vi "总磷插入数据.vi"(0 "table":string, 5 "data":T2={"时间标识"=timestamp(0 s since 1904-01-01), "测量模式"=enum."水样测试", "数据标记表"="N", "监测值"=0.0, "单位"=0, "数据标识"="", "因子编码"=0, "标样参考值"=0.0, "F0"=0.0, "F1"=0.0, "F2"=0.0, "F3"=0.0, "F4"=0.0, "F5"=0.0, "F6"=0.0, "F7"=0.0, "X"=0.0, "温度"=0.0, "湿度"=0.0, "量程标识"="", "SN"=""} {"单位" items=["μg/L", "mg/L", "ppm", "mg/m3", "cm", "ppb", "μg/m3", "%", "nmol/mol", "μmol/mol", "MPN/L", "MPN/100ml", "ng/m3", "NTU", "无量纲", "ms/cm", "μs/cm"]}, 11 "error in (no error)":errorcluster) -> (15 "error out":errorcluster)   [LabVIEW 2016, in "斯坦道总磷.lvlib"]
uses:
  <vilib>/Utility/sysdir.llb/System Directory Type.ctl
  <vilib>/Utility/error.llb/DialogType.ctl
  <vilib>/addons/database/Auxilliary.llb/DB Tools Column Info.ctl
  <vilib>/addons/database/Auxilliary.llb/DB Tools DataTypes.ctl
  <vilib>/addons/database/Connection.llb/DB Tools Open Connec (String).vi
  <vilib>/addons/database/Connection.llb/Conn Execute.vi
  <vilib>/addons/database/Recordset.llb/Rec Fetch Recordset Data (R).vi
  <vilib>/addons/database/Recordset.llb/Rec Destroy - Connection.vi
  <vilib>/addons/database/NI_Database_API.lvlib
  WxMessage/wxpusher.lvlib
panel:
  out "data修正输出":T1
  out "data输出":T1
  out "为空？":bool
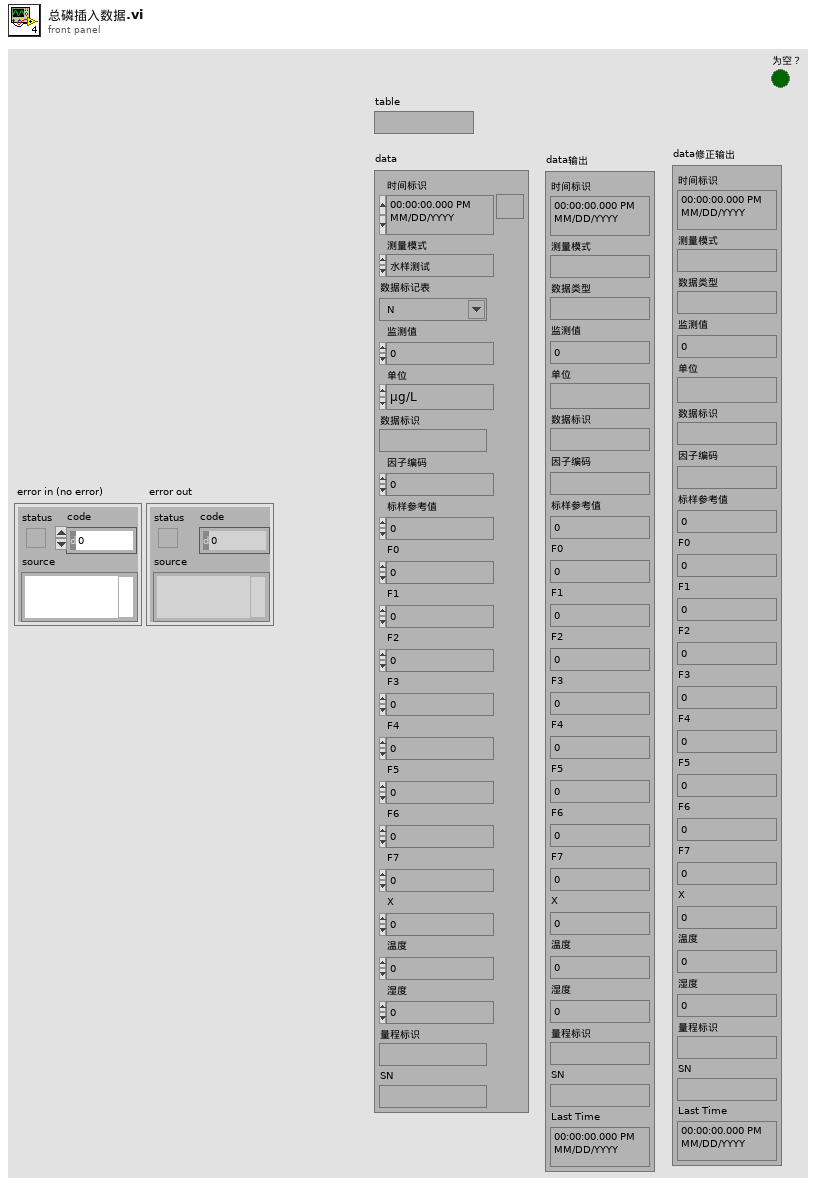
[diagram p1: front panel]
types:
  T1 = cluster{"时间标识":timestamp, "测量模式":string, "数据类型":string, "监测值":sgl, "单位":string, "数据标识":string, "因子编码":string, "标样参考值":sgl, "F0":sgl, "F1":sgl, "F2":sgl, "F3":sgl, "F4":sgl, "F5":sgl, "F6":sgl, "F7":sgl, "X":sgl, "温度":sgl, "湿度":sgl, "量程标识":string, "SN":string, "Last Time":timestamp}
  T2 = cluster{"时间标识":timestamp, "测量模式":enum16{"维护数据", "水样测试", "标样核查", "零点核查", "跨度核查", "空白测试", "平行样测试", "加标回收", "空白校准", "标样校准", "初始化（清洗）"}, "数据标记表":string, "监测值":sgl, "单位":u16, "数据标识":string, "因子编码":u32, "标样参考值":sgl, "F0":sgl, "F1":sgl, "F2":sgl, "F3":sgl, "F4":sgl, "F5":sgl, "F6":sgl, "F7":sgl, "X":sgl, "温度":sgl, "湿度":sgl, "量程标识":string, "SN":string}
  T3 = typedef "DialogType.ctl" = u16
  T4 = typedef "System Directory Type.ctl" = i32
  T5 = typedef "NI_Database_API.lvlib/Conn ObjectReference.ctl" = refnum<k1>
  T6 = typedef "NI_Database_API.lvlib/Rec ObjectReference.ctl" = refnum<k1>
  T7 = typedef "NI_Database_API.lvlib/DB Tools Column Info.ctl" = cluster{"column name":string, "data type":T8, "size":i32, "allow null?":bool}
  T8 = typedef "NI_Database_API.lvlib/DB Tools DataTypes.ctl" = enum16{"String", "Long (I32)", "Single (SGL)", "Double (DBL)", "Date/Time", "Binary"}
  T9 = cluster{"切换阈值":dbl, "稳定系数":dbl, "变异系数":dbl, "enable":bool, "init":bool}
  T10 = cluster{"数值输出":dbl, "均值":dbl, "变异系数":dbl, "数据波动百分比":dbl, "随机数flag":bool}
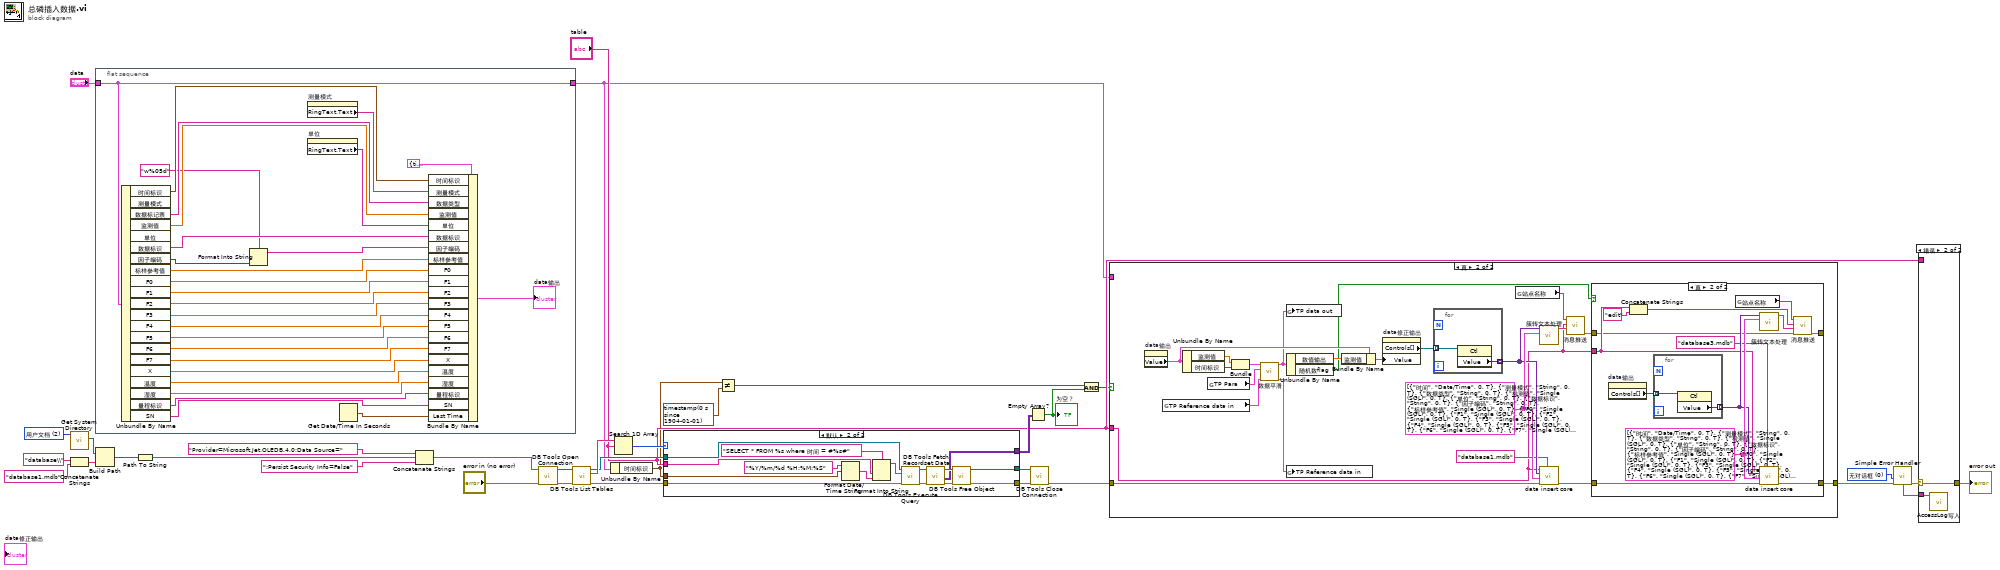
[diagram p0: block diagram]
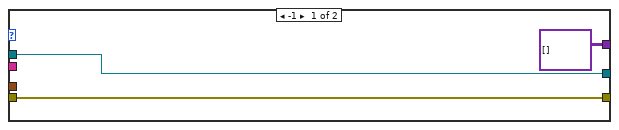
[diagram p5: hidden frame]
diagram:
  w16 = T3 0 items=["无对话框", "确定信息", "继续或停止信息", "确定信息＋警告", "继续/停止+警告"] ("type of dialog (OK msg:1)")
  w33 = T4 2 items=["用户目录"=0, "用户桌面"=1, "用户文档"=2, "用户应用程序数据"=3, "用户设置"=4, "用户临时目录"=5, "公共文档"=6, "公共应用程序数据"=7, "公共设置"=8, "公共缓存"=13, "系统核心库"=9, "系统安装库"=10, "应用程序文件"=11, "启动盘根目录"=12] ("system directory type")
  n1 = call <vilib>:"Get System Directory.vi"("system directory type"=w33) -> ("system directory"=w31:path)  [unwired: 10 in]
  n2 = Concatenate Strings("database\\" ("condition"), "database1.mdb" ("字符串")) -> (w25:string)
  n3 = flat-sequence {
    tunnel: "data" -> [w38]
    tunnel: [w38] -> w10
    frame #0 {
      n4 = Unbundle By Name(w38) -> ("时间标识"=w59:timestamp, "数据标记表"=w57:string, "监测值"=w56:sgl, "数据标识"=w54:string, "因子编码"=w37:u32, "标样参考值"=w53:sgl, "F0"=w52:sgl, "F1"=w51:sgl, "F2"=w50:sgl, "F3"=w49:sgl, "F4"=w48:sgl, "F5"=w47:sgl, "F6"=w46:sgl, "F7"=w45:sgl, "X"=w44:sgl, "温度"=w43:sgl, "湿度"=w42:sgl, "量程标识"=w41:string, "SN"=w40:string)  [unwired: 2 out]
      n5 = Format Into String(format string="w%05d" ("格式字符串"), w37) -> (resulting string=w35:string)  [unwired: 2 in, 1 out]
      n6 = property on="测量模式" class="Enum (严格)"() -> ("RingText.Text"=w58:string)  [unwired: 2 in, 2 out]
      n7 = property on="单位" class="Ring (严格)"() -> ("RingText.Text"=w55:string)  [unwired: 2 in, 2 out]
      n8 = Get Date/Time In Seconds() -> (seconds since 1Jan1904=w39:timestamp)
      n9 = Bundle By Name(cluster=T1 {"时间标识"=timestamp(0 s since 1904-01-01), "测量模式"="", "数据类型"="", "监测值"=0.0, "单位"="", "数据标识"="", "因子编码"="", "标样参考值"=0.0, "F0"=0.0, "F1"=0.0, "F2"=0.0, "F3"=0.0, "F4"=0.0, "F5"=0.0, "F6"=0.0, "F7"=0.0, "X"=0.0, "温度"=0.0, "湿度"=0.0, "量程标识"="", "SN"="", "Last Time"=timestamp(0 s since 1904-01-01)} ("data输出"), "时间标识"=w59, "测量模式"=w58, "数据类型"=w57, "监测值"=w56, "单位"=w55, "数据标识"=w54, "因子编码"=w35, "标样参考值"=w53, "F0"=w52, "F1"=w51, "F2"=w50, "F3"=w49, "F4"=w48, "F5"=w47, "F6"=w46, "F7"=w45, "X"=w44, "温度"=w43, "湿度"=w42, "量程标识"=w41, "SN"=w40, "Last Time"=w39) -> (→"data输出":T1)
    }
  }
  n10 = Build Path(base path=w31, name or relative path=w25) -> (appended path=w30:path)
  n11 = Path To String(path=w30) -> (string=w29:string)
  n12 = Concatenate Strings("Provider=Microsoft.Jet.OLEDB.4.0;Data Source=" ("condition"), w29, ";Persist Security Info=False" ("condition")) -> (w27:string)
  n13 = call-poly <vilib>:"DB Tools Open Connection.vi"("error in (no error)"="error in (no error)", "connection information"=w27) -> ("error out"=w22:errorcluster, "connection reference"=w23:T5)  [unwired: 6 in]
  n14 = call <vilib>:"DB Tools List Tables.vi"("error in (no error)"=w22, "connection reference"=w23) -> ("error out"=w17:errorcluster, "tables"=w21:string[], "connection reference out"=w18:T5)  [unwired: 3 in]
  n15 = Unbundle By Name(w10) -> ("时间标识"=w6:timestamp)
  n16 = Search 1D Array(1D array=w21, element="table") -> (index of element=w20:i32)  [unwired: 1 in]
  n17 = case shown="默认" w20 {
    tunnel: [variant[][] [] ("recordset data") w75] -> w24
    tunnel: [w64 w74] -> w5
    tunnel: [w63 w73] -> w4
    tunnel: w18 -> [w64 w69]
    tunnel: w17 -> [w63 w68]
    tunnel: "table" -> [_ w67]
    tunnel: w6 -> [_ w65]
    frame -1 {
    }
    frame Default {
      n18 = Format Date/Time String(time format string (%c)="%Y/%m/%d %H:%M:%S" ("时间格式字符串(%c)"), seconds (now)=w65) -> (date/time string=w70:string)  [unwired: 1 in]
      n19 = Format Into String(format string="SELECT * FROM %s where 时间 = #%s#" ("格式字符串"), w67, w70) -> (resulting string=w72:string)  [unwired: 2 in, 1 out]
      n20 = call-poly <vilib>:"DB Tools Execute Query.vi"("error in (no error)"=w68, "SQL query"=w72, "connection reference"=w69) -> ("error out"=w76:errorcluster, "recordset reference"=w79:T6)  [unwired: 5 in]
      n21 = call-poly <vilib>:"DB Tools Fetch Recordset Data.vi"("error in (no error)"=w76, "recordset reference"=w79) -> ("error out"=w77:errorcluster, "recordset data"=w75:variant[][], "recordset reference out"=w78:T6)  [unwired: 3 in]
      n22 = call-poly <vilib>:"DB Tools Free Object.vi"("error in (no error)"=w77, "recordset reference"=w78) -> ("error out"=w73:errorcluster, "connection reference"=w74:T5)  [unwired: 8 in]
    }
  }
  n23 = Not Equal?(x=w6, y=timestamp(0 s since 1904-01-01)) -> (x != y?=w7:bool)
  n24 = Empty Array?(array=w24) -> (empty?=w19:bool)
  "为空？" <- w19
  n25 = call <vilib>:"DB Tools Close Connection.vi"("error in (no error)"=w4, "connection reference"=w5) -> ("error out"=w3:errorcluster)  [unwired: 5 in]
  n26 = And(x=w7, y=w19) -> (x .and. y?=w8:bool)
  n27 = case shown="真" w8 {
    tunnel: "table" -> [_ w82]
    tunnel: w10 -> [_ _]
    tunnel: w3 -> [w80 w102]
    tunnel: [w80 w83] -> w2
    frame False {
    }
    frame True {
      w100 = T7[] [{"column name"="时间", "data type"=enum."Date/Time", "size"=0, "allow null?"=TRUE}, {"column name"="测量模式", "data type"=enum."String", "size"=0, "allow null?"=TRUE}, {"column name"="数据类型", "data type"=enum."String", "size"=0, "allow null?"=TRUE}, {"column name"="检测值", "data type"=enum."Single (SGL)", "size"=0, "allow null?"=TRUE}, {"column name"="单位", "data type"=enum."String", "size"=0, "allow null?"=TRUE}, {"column name"="数据标识", "data type"=enum."String", "size"=0, "allow null?"=TRUE}, {"column name"="因子编码", "data type"=enum."String", "size"=0, "allow null?"=TRUE}, {"column name"="标样参考值", "data type"=enum."Single (SGL)", "size"=0, "allow null?"=TRUE}, {"column name"="F0", "data type"=enum."Single (SGL)", "size"=0, "allow null?"=TRUE}, {"column name"="F1", "data type"=enum."Single (SGL)", "size"=0, "allow null?"=TRUE}, {"column name"="F2", "data type"=enum."Single (SGL)", "size"=0, "allow null?"=TRUE}, {"column name"="F3", "data type"=enum."Single (SGL)", "size"=0, "allow null?"=TRUE}, {"column name"="F4", "data type"=enum."Single (SGL)", "size"=0, "allow null?"=TRUE}, {"column name"="F5", "data type"=enum."Single (SGL)", "size"=0, "allow null?"=TRUE}, {"column name"="F6", "data type"=enum."Single (SGL)", "size"=0, "allow null?"=TRUE}, {"column name"="F7", "data type"=enum."Single (SGL)", "size"=0, "allow null?"=TRUE}, {"column name"="X", "data type"=enum."Single (SGL)", "size"=0, "allow null?"=TRUE}, {"column name"="温度", "data type"=enum."Single (SGL)", "size"=0, "allow null?"=TRUE}, {"column name"="湿度", "data type"=enum."Single (SGL)", "size"=0, "allow null?"=TRUE}, {"column name"="量程标识", "data type"=enum."String", "size"=0, "allow null?"=TRUE}, {"column name"="SN", "data type"=enum."String", "size"=0, "allow null?"=TRUE}, {"column name"="LastTime", "data type"=enum."Date/Time", "size"=0, "allow null?"=TRUE}] ("column information")
      n28 = property on="data输出" class="Clust (严格)"() -> ("Value"=w90:T1)  [unwired: 2 in, 2 out]
      n29 = global read "仿真全局变量.vi" "TP Reference data in"() -> (w96:cluster{"参考数值":dbl[], "参考数值时间戳":timestamp[]})
      n30 = Unbundle By Name(w90) -> ("监测值"=w93:sgl, "时间标识"=w94:timestamp)
      n31 = global read "仿真全局变量.vi" "TP Para"() -> (w95:T9)
      n32 = Bundle("监测值"=w93, "时间标识"=w94) -> (w92:cluster{"监测值":sgl, "时间标识":timestamp})  [unwired: 1 in]
      n33 = call "数据平滑.vi"("Reference data in"=w96, "Para"=w95, "data in"=w92) -> ("Reference data out"=w97:cluster{"参考数值":dbl[], "参考数值时间戳":timestamp[]}, "data out"=w89:T10)  [unwired: 7 in]
      n34 = global write "仿真全局变量.vi" "TP data out"(w89) -> ()
      n35 = Unbundle By Name(w89) -> ("数值输出"=w88:dbl, "随机数flag"=w85:bool)
      n36 = global write "仿真全局变量.vi" "TP Reference data in"(w97) -> ()
      n37 = Bundle By Name(cluster=w90, "监测值"=w88) -> (w87:T1)
      n38 = property on="data修正输出" class="Clust (严格)"("Value"=w87) -> ("Controls[]"=w91:refnum<vi>[])  [unwired: 2 in, 2 out]
      n39 = for {
        tunnel: w91 -> [w120] mode=indexing
        tunnel: [w119] -> w99 mode=indexing
        n40 = property class="Ctl"(reference=w120) -> ("Value"=w119:variant)  [unwired: 1 in, 2 out]
      }
      n41 = global read "系统设置全局变量.vi" "站点名称"() -> (w98:string)
      n42 = call "簇转文本处理.vi"("column information"=w100, "data"=w99) -> ("output"=w101:string)  [unwired: 9 in]
      n43 = call "data insert core.vi"("database"="database1.mdb", "error in (no error)"=w102, "column information"=w100, "data"=w99, "table"=w82) -> ("error out"=w84:errorcluster)  [unwired: 6 in]
      n44 = call "消息推送.vi"("数据内容"=w101, "参数"=w82, "站点"=w98) -> ("error out"=w81:errorcluster)  [unwired: 8 in]
      n45 = case shown="真" w85 {
        tunnel: w84 -> [w103 w110]
        tunnel: [w103 w109] -> w83
        tunnel: w82 -> [_ w108]
        tunnel: w81 -> [_ w105]
        tunnel: [_ w104] -> _
        frame False {
        }
        frame True {
          w115 = T7[] [{"column name"="时间", "data type"=enum."Date/Time", "size"=0, "allow null?"=TRUE}, {"column name"="测量模式", "data type"=enum."String", "size"=0, "allow null?"=TRUE}, {"column name"="数据类型", "data type"=enum."String", "size"=0, "allow null?"=TRUE}, {"column name"="检测值", "data type"=enum."Single (SGL)", "size"=0, "allow null?"=TRUE}, {"column name"="单位", "data type"=enum."String", "size"=0, "allow null?"=TRUE}, {"column name"="数据标识", "data type"=enum."String", "size"=0, "allow null?"=TRUE}, {"column name"="因子编码", "data type"=enum."String", "size"=0, "allow null?"=TRUE}, {"column name"="标样参考值", "data type"=enum."Single (SGL)", "size"=0, "allow null?"=TRUE}, {"column name"="F0", "data type"=enum."Single (SGL)", "size"=0, "allow null?"=TRUE}, {"column name"="F1", "data type"=enum."Single (SGL)", "size"=0, "allow null?"=TRUE}, {"column name"="F2", "data type"=enum."Single (SGL)", "size"=0, "allow null?"=TRUE}, {"column name"="F3", "data type"=enum."Single (SGL)", "size"=0, "allow null?"=TRUE}, {"column name"="F4", "data type"=enum."Single (SGL)", "size"=0, "allow null?"=TRUE}, {"column name"="F5", "data type"=enum."Single (SGL)", "size"=0, "allow null?"=TRUE}, {"column name"="F6", "data type"=enum."Single (SGL)", "size"=0, "allow null?"=TRUE}, {"column name"="F7", "data type"=enum."Single (SGL)", "size"=0, "allow null?"=TRUE}, {"column name"="X", "data type"=enum."Single (SGL)", "size"=0, "allow null?"=TRUE}, {"column name"="温度", "data type"=enum."Single (SGL)", "size"=0, "allow null?"=TRUE}, {"column name"="湿度", "data type"=enum."Single (SGL)", "size"=0, "allow null?"=TRUE}, {"column name"="量程标识", "data type"=enum."String", "size"=0, "allow null?"=TRUE}, {"column name"="SN", "data type"=enum."String", "size"=0, "allow null?"=TRUE}, {"column name"="LastTime", "data type"=enum."Date/Time", "size"=0, "allow null?"=TRUE}] ("column information")
          n46 = property on="data输出" class="Clust (严格)"() -> ("Controls[]"=w112:refnum<vi>[])  [unwired: 2 in, 2 out]
          n47 = Concatenate Strings(w108, "edit" ("字符串")) -> (w107:string)
          n48 = for {
            tunnel: w112 -> [w118] mode=indexing
            tunnel: [w117] -> w114 mode=indexing
            n49 = property class="Ctl"(reference=w118) -> ("Value"=w117:variant)  [unwired: 1 in, 2 out]
          }
          n50 = global read "系统设置全局变量.vi" "站点名称"() -> (w113:string)
          n51 = call "簇转文本处理.vi"("column information"=w115, "data"=w114) -> ("output"=w116:string)  [unwired: 9 in]
          n52 = call "data insert core.vi"("database"="database3.mdb", "error in (no error)"=w110, "column information"=w115, "data"=w114, "table"=w108) -> ("error out"=w109:errorcluster)  [unwired: 6 in]
          n53 = call "消息推送.vi"("error in (no error)"=w105, "数据内容"=w116, "参数"=w107, "站点"=w113) -> ("error out"=w104:errorcluster)  [unwired: 7 in]
        }
      }
    }
  }
  n54 = call <vilib>:"Simple Error Handler.vi"("type of dialog (OK msg:1)"=w16, "error in (no error)"=w2) -> ("error out"=w15:errorcluster, "message"=w14:string)  [unwired: 3 in, 3 out]
  n55 = case shown="错误" w15 {
    selector: w15 -> [_ w121]
    tunnel: w14 -> [_ w122]
    tunnel: [_ w121] -> w13
    tunnel: "table" -> [_ _]
    frame No Error {
    }
    frame Error {
      n56 = call "AccessLog写入.vi"("Log"=w122) -> ()  [unwired: 11 in]
    }
  }
  "error out" <- w13
